vi "Nicolet 12 ICAI_gatefix2.vi"(3 "?":u16(ring)=9 items=["16", "32", "64", "128", "256", "512", "1024", "2048", "4096", "8192", "16384", "32768", "65536", "131072", "262144", "524288 (one channel)", ""], 5 "Sample Duration (sec)":u32(knob)=24 scale=1.0..33.0) -> (0 "Waveform Graph":waveform(dbl)[](graph)=[{"t0"=timestamp(0 s since 1904-01-01), "dt"=0.0001220703125, "Y"=array[40960 elements]}, {"t0"=timestamp(0 s since 1904-01-01), "dt"=0.0001220703125, "Y"=array[40960 elements]}], 2 "data":dbl[][](array[numeric]) format="%0.2f", 8 "points":i32=40960)   [LabVIEW 2010]
doc: "I. Description:\nThis example demonstrates how to acquire a finite amount of data (Waveform) using the DAQ device's internal clock, started by an analog edge condition.\n\nII. Instructions for Running:\n1. Select the physical channel to correspond to where your signal is input on the DAQ device.\n2. Enter the minimum and maximum voltage range.\nNote: For better accuracy try to match the input range to the expected voltage level of the measured signal.\n3. Set the number of samples to acquire per channel.\n4. Set the rate of the acquisition\nNote: The rate should be AT LEAST twice as fast as the maximum frequency component of the signal being acquired.\n5. Set the source of the start trigger. By default this is PFI0\n6. Set the slope and level of desired analog edge condition.\n\nIII. Block Diagram Steps:\n1. Create an empty task.\n2. Create an analog input voltage channel.\n3. Set the rate for the sample clock. Additionally, define the sample mode to be finite.\n4. Define the parameters for an Analog Slope Start Trigger.\n5. Call the Start VI to start the acquisition.\n6. Read all of the data.\n7. Stop the Analog Input Task.\n8. Call the Clear Task VI to clear the Task.\n9. Use the popup dialog box to display an error if any\nIV. I/O Connections Overview:\nMake sure your signal input terminal matches the Physical Channel I/O Control. In this case wire your signal to the ai0 pin on your DAQ Device."
uses:
  programs/Detection/200262.llb/Trigger Select.ctl
  <vilib>/Utility/error.llb/DialogType.ctl
  <vilib>/DAQmx/write.llb/DAQmx Write (Analog DBL 1Chan 1Samp).vi
  <vilib>/DAQmx/read.llb/DAQmx Read (Analog 2D DBL NChan NSamp).vi
  <vilib>/DAQmx/create/channels.llb/DAQmx Create Channel (AO-Voltage-Basic).vi
  <vilib>/daqmx/miscellaneous.llb/DAQmx Fill In Error Info.vi
  <vilib>/DAQmx/create/channels.llb/DAQmx Create Channel (AI-Voltage-Basic).vi
  <vilib>/DAQmx/configure/timing.llb/DAQmx Timing (Sample Clock).vi
  <vilib>/DAQmx/configure/trigger.llb/DAQmx Start Trigger (Analog Edge).vi
  <vilib>/DAQmx/configure/trigger.llb/DAQmx Reference Trigger (Digital Edge).vi
  <vilib>/measure/maspectr.llb/FFT Power Spectral Density for 1 Chan.vi
  <vilib>/measure/NI_MAPro.lvlib
  Program Files/National Instruments/LabVIEW 2010/resource/objmgr/daqmx.rc
panel:
  out "size(s)":i32[](array[numeric])
  in  "CAI/ICAI":bool=TRUE
  in  "?":path=path "C:/Users/Cardenas/Desktop/7_01/7_01_380fringe371mvmid_lockedat330.txt"
  in  "Path":path=path "C:/Users/Cardenas/Desktop/7_03/a6_200ms_span.txt"
  out "Time":dbl=5.5
  out "points pretriger":dbl=4096.0
  in  "Iterations to Average":i32=30
  in  "Sample Rate Hz":bool
  out "Cursor Time Selected":dbl=0.22413589186805782
  out "Cursor Peak to Peak Voltage":dbl=0.01024955436720143
  in  "Save Average To File":bool
  out "Pretrigger Samples":dbl=4096.0
  out "Seconds Per Division":dbl=0.1
  out "Posttrigger Samples Captured":dbl=40960.0
  in  "Voltage Offset":dbl(knob) scale=-2.0..2.0
  in  "Average / Live Display":bool
  in  "Seconds  Per Division":u32(knob) min=1 max=1 step=1 scale=0.0..15.0
  out "Samples Averaged":i32=3
  in  "?":bool=TRUE
  in  "Volts Per Division":dbl(knob)=0.5 scale=0.005..5.0
  in  "Pretrigger Duration (%)":dbl(knob)=0.1 min=0.0 max=2.0 step=1.0 scale=0.05..0.95
  in  "Analog Source":string="APFI0"
  in  "Digital External TTL Source":tag="/Dev1/PFI0"
  in  "Trigger Type":T1=enum."Analog Edge"
  in  "Analog Edge Level":dbl=-0.1 format="%0.2f"
  in  "Edge":i32(ring)=10280 items=["Rising"=10280, "Falling"=10171]
  in  "Physical Channel":tag="Dev1/ai22, Dev1/ai23" caption="Physical Channels"
  out "Sampling Iterations":i32=2
  in  "Maximum  Voltage":dbl=10.0
  in  "Minimum Voltage":dbl=-10.0
  out "Sampling Rate":i32=8192 caption="Sample Rate (Hz)"
  in  "stop":bool
  # "Channel\nConfiguration"
  # "Triggering Parameters"
  # "Voltage Parameters"
  # "TTL Trigger Options"
  # "Timing Parameters"
  # "External  Trigger Options"
  # "Storage Options"
  # "Nicolet 8.vi*If X scale markers are not drawn:\nRight click the waveform diagram -> select X axis -> marker spacing -> set to arbitrary AFTER\nsetting the correct seconds per division"
  # "CAI / ICAI"
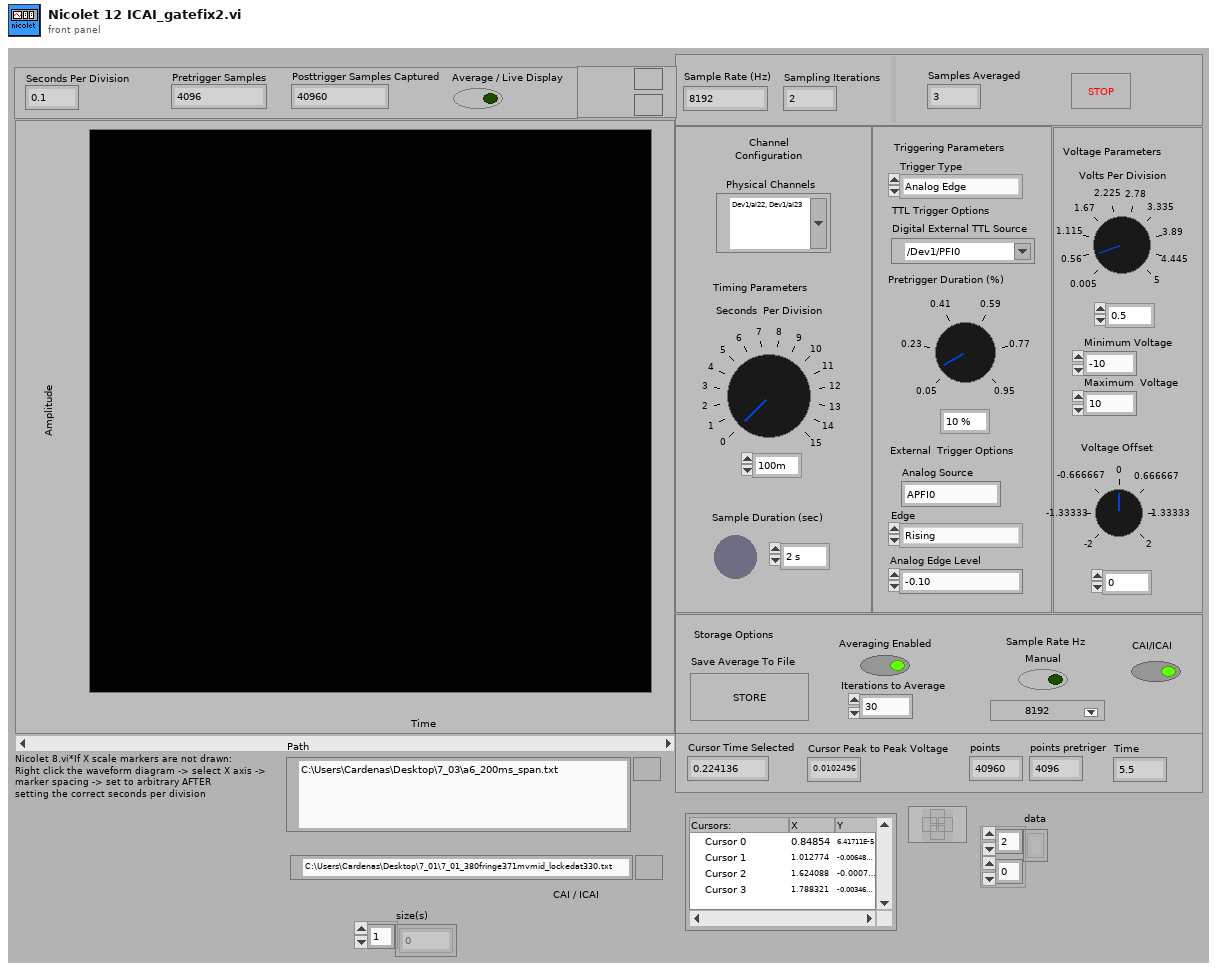
[diagram p1: front panel]
types:
  T1 = typedef "Trigger Select.ctl" = enum16{"None", "Analog Edge", "Digital Edge"}
  T2 = typedef "DialogType.ctl" = u16
  T3 = typedef "LVCursorListTypeDef.ctl" = cluster{"Name":string, "Color":u32, "Style":u8, "Point Style":u8, "Name Visible":bool, "Allow Drag":bool, "Cursor Mode":u32, "Plot":i32, "Index":i32, "Position":cluster{"X":dbl, "Y":dbl}, "X Scale":u32, "Y Scale":u32, "Watch Plots":i32[], "Watch All Plots":bool, "Plot Area":i32, "Label Offset":cluster{"X":dbl, "Y":dbl}}[]
  T4 = cluster{"Name":string, "Color":u32, "Style":u8, "Point Style":u8, "Name Visible":bool, "Allow Drag":bool, "Cursor Mode":u32, "Plot":i32, "Index":i32, "Position":cluster{"X":dbl, "Y":dbl}, "X Scale":u32, "Y Scale":u32, "Watch Plots":i32[], "Watch All Plots":bool, "Plot Area":i32, "Label Offset":cluster{"X":dbl, "Y":dbl}}
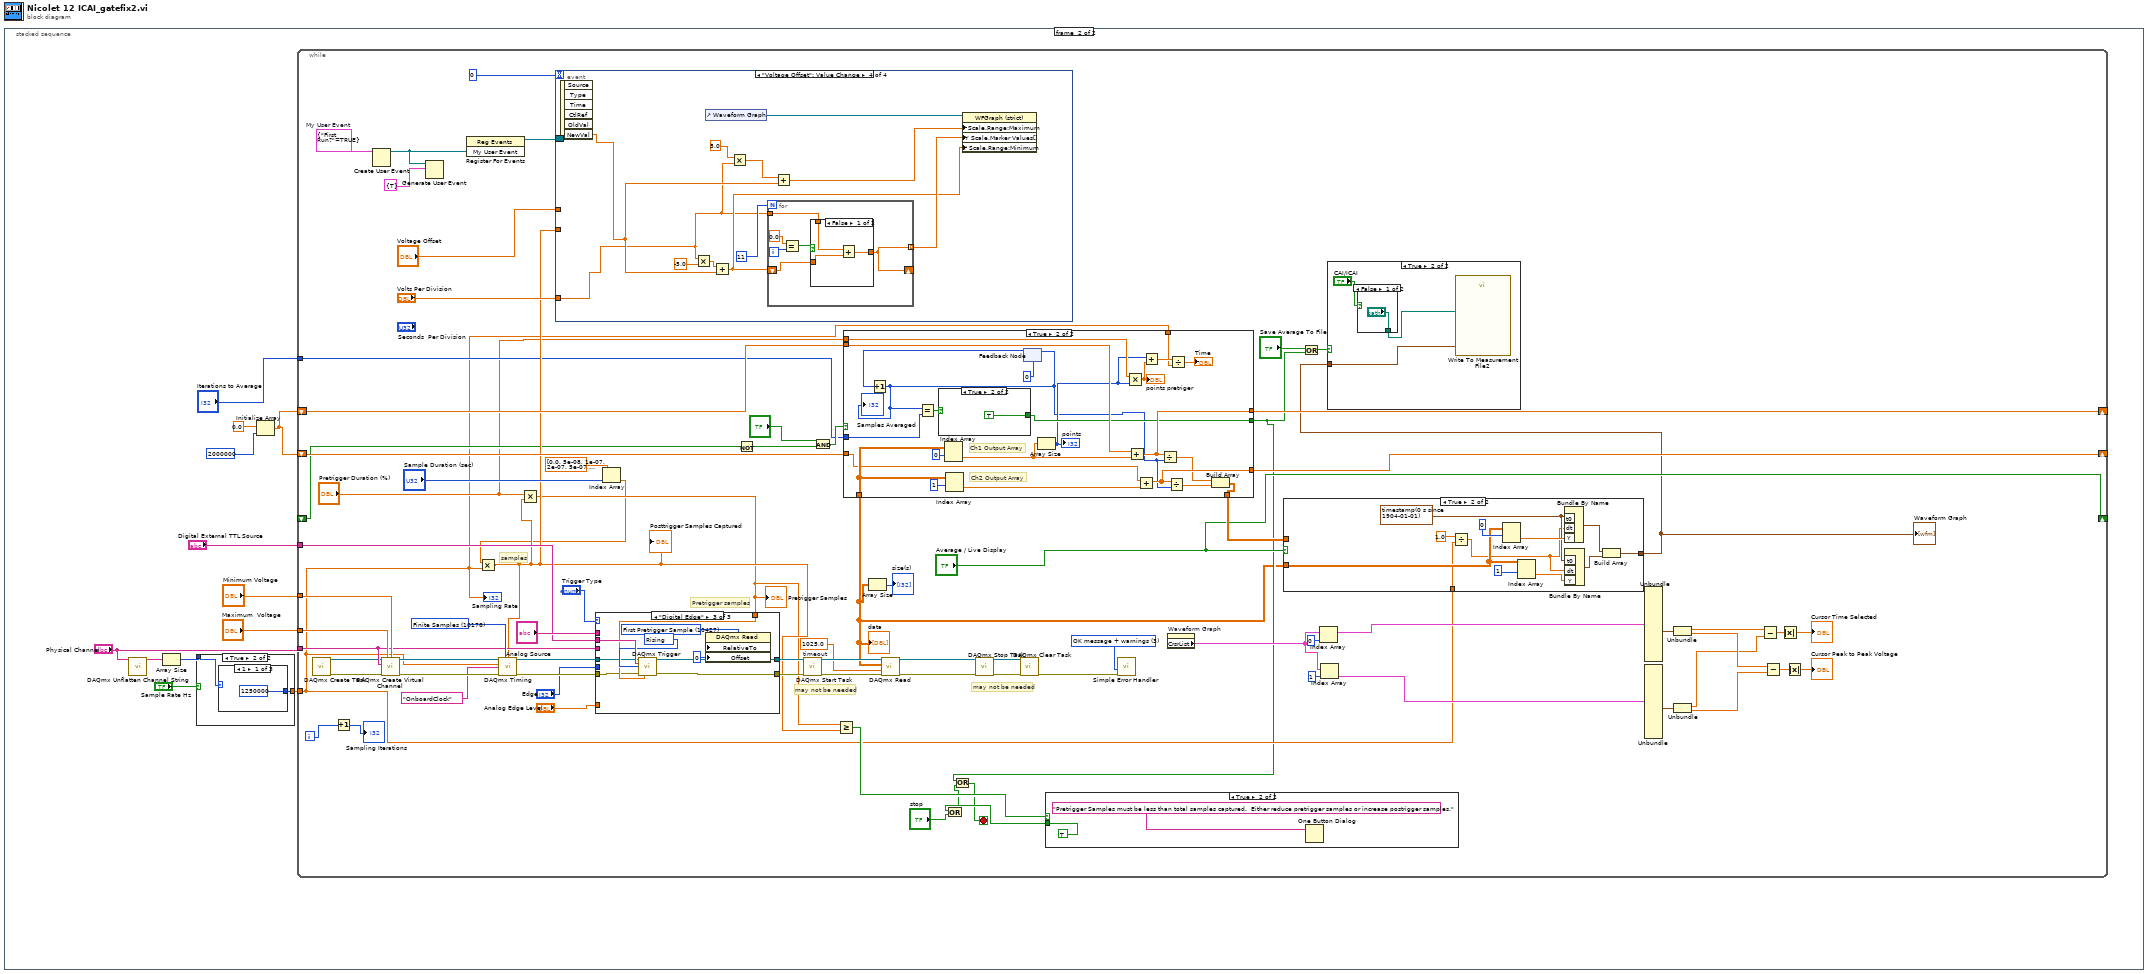
[diagram p0: block diagram]
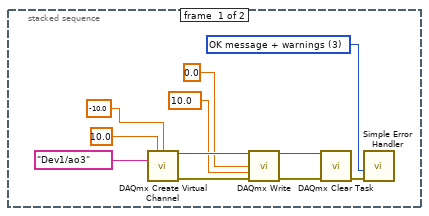
[diagram p2: hidden frame]
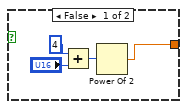
[diagram p3: hidden frame]
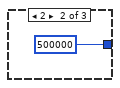
[diagram p4: hidden frame]
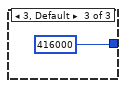
[diagram p5: hidden frame]
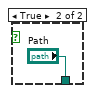
[diagram p7: hidden frame]
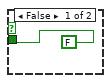
[diagram p8: hidden frame]
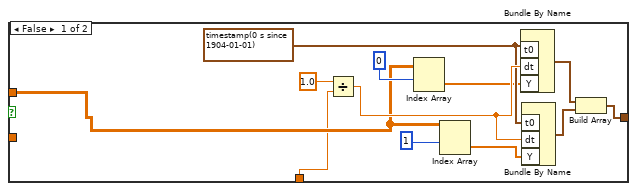
[diagram p9: hidden frame]
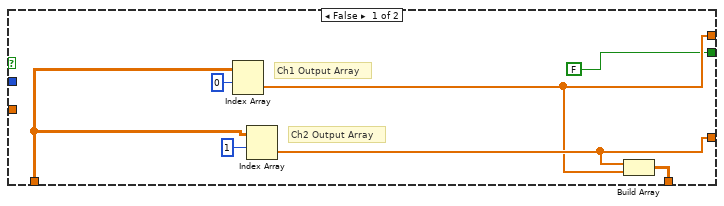
[diagram p10: hidden frame]
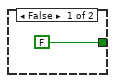
[diagram p11: hidden frame]
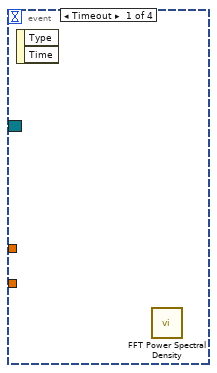
[diagram p12: hidden frame]
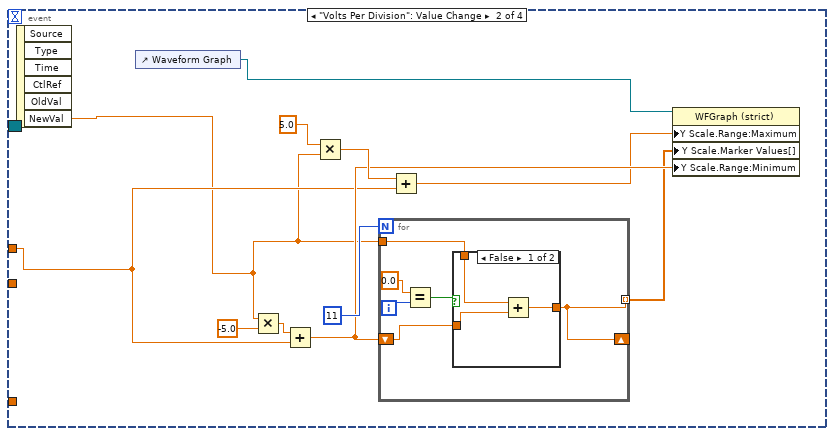
[diagram p13: hidden frame]
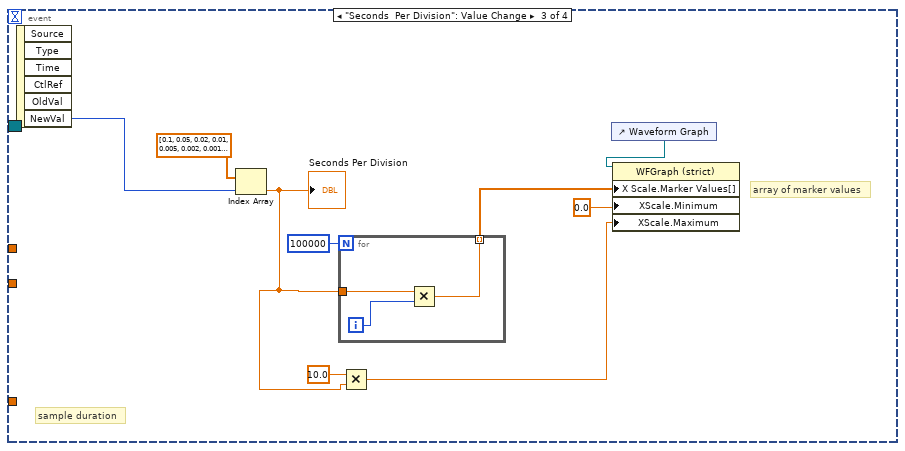
[diagram p15: hidden frame]
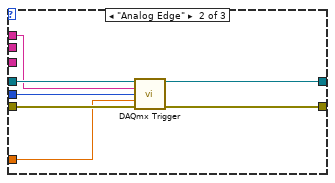
[diagram p18: hidden frame]
diagram:
  n1 = stacked-sequence {
    frame #0 {
      w4 = T2 3 items=["no dialog", "OK message", "continue or stop message", "OK message + warnings", "continue/stop + warnings"] ("type of dialog (OK msg:1)")
      n2 = call-poly <vilib>:"DAQmx Create Virtual Channel.vi"("maximum value"=10.0 ("Maximum Value"), "minimum value"=-10.0 ("Minimum Value"), "physical channels"=tag "Dev1/ao3" ("Physical Channel")) -> ("task out"=w7:refnum<k21>, "error out"=w8:errorcluster)  [unwired: 6 in, 5 out]
      n3 = call-poly <vilib>:"DAQmx Write.vi"("task/channels in"=w7, "data"=0.0 ("Voltage Output"), "timeout"=10.0, "error in"=w8) -> ("task out"=w2:refnum<k21>, "error out"=w3:errorcluster)  [unwired: 1 in, 9 out]
      n4 = call <vilib>:"DAQmx Clear Task.vi"("task in"=w2, "error in"=w3) -> ("error out"=w1:errorcluster)  [unwired: 13 out]
      n5 = call <vilib>:"Simple Error Handler.vi"("type of dialog (OK msg:1)"=w4, "error in (no error)"=w1) -> ()  [unwired: 8 out]
    }
    frame #1 {
      n6 = call <vilib>:"DAQmx Unflatten Channel String.vi"("names in"="Physical Channel") -> ("names out"=w19:string[])  [unwired: 1 in, 13 out]
      n7 = Array Size(array=w19) -> (size(s)=w17:i32)
      n8 = case shown="True" "Sample Rate Hz" {
        tunnel: [w25 w29] -> w18
        tunnel: w17 -> [_ w28]
        frame False {
          n9 = Add(x=4, y="?") -> (x+y=w26:i32)
          n10 = Power Of 2(x=w26) -> (2^x=w25:dbl)
        }
        frame True {
          n11 = case shown="1" w28 {
            tunnel: [1250000 500000 416000] -> w29
            frame 1 {
            }
            frame 2 {
            }
            frame 3, Default {
            }
          }
        }
      }
      n12 = Initialize Array(0.0, 2000000) -> (w12:dbl[])
      n13 = while {
        tunnel: "Minimum Voltage" -> [w93]
        tunnel: "Maximum  Voltage" -> [w92]
        tunnel: "Physical Channel" -> [w91]
        tunnel: "Digital External TTL Source" -> [w89]
        shift-right: [w83] -> _
        shift-left: w12 -> [w82]
        shift-right: [w78] -> _
        shift-left: w12 -> [w77]
        tunnel: w18 -> [w40]
        shift-right: ["Average / Live Display"] -> _
        shift-left: _ -> [w50]
        tunnel: "Iterations to Average" -> [w42]
        i -> [w36]
        stop <- w39 stop-if-true
        w88 = cluster{"First Run?":bool} {"First Run?"=TRUE}  # My User Event
        w108 = T2 3 items=["no dialog", "OK message", "continue or stop message", "OK message + warnings", "continue/stop + warnings"] ("type of dialog (OK msg:1)")
        w105 = 1025.0  # timeout
        w103 = 10178 items=["Finite Samples"=10178, "Continuous Samples"=10123] ("sample mode")
        # "samples"
        # "may not be needed"
        # "may not be needed"
        # "Pretrigger samples"
        n14 = call <vilib>:"DAQmx Create Task.vi"() -> ("task out"=w81:refnum<k21>, "error out"=w80:errorcluster)  [unwired: 5 in, 9 out]
        n15 = Increment(x=w36) -> (x+1=→"Sampling Iterations":i32)
        n16 = Create User Event(user event datatype=w88) -> (user event=w86:refnum<user-event>)  [unwired: 1 in, 1 out]
        n17 = call-poly <vilib>:"DAQmx Create Virtual Channel.vi"("task in"=w81, "maximum value"=w92, "minimum value"=w93, "physical channels"=w91, "error in"=w80) -> ("task out"=w104:refnum<k21>, "error out"=w112:errorcluster)  [unwired: 4 in, 5 out]
        n18 = Generate User Event(user event=w86, event data cluster=cluster{"First Run?":bool} {"First Run?"=TRUE} ("event data")) -> ()  [unwired: 1 in, 2 out]
        n19 = register-events(w86) -> (reference out=w84:refnum<event-registration>)  [unwired: 2 in, 1 out]
        n20 = Index Array(array=dbl[] [0.0, 5e-08, 1e-07, 2e-07, 5e-07, 1e-06, 2e-06, 5e-06, 1e-05, 2e-05, 5e-05, 0.0001, 0.0002, 0.0005, 0.001, 0.002, 0.005, 0.01, 0.02, 0.05, 0.1, 0.2, 0.5, 1.0, 2.0, 5.0, 10.0, 16.5, 32.5, 65.0, 129.0, 257.0, 513.0, 1025.0], index="Sample Duration (sec)") -> (element=w47:dbl)
        n21 = Multiply(x=w47, y=w40) -> (x*y=w69:dbl)
        "Posttrigger Samples Captured" <- w69
        n22 = call-poly <vilib>:"DAQmx Timing.vi"("task/channels in"=w104, "sample mode"=w103, "samples per channel"=w69, "rate"=w40, "source"=tag "OnboardClock", "error in"=w112) -> ("task out"=w98:refnum<k21>, "error out"=w96:errorcluster)  [unwired: 1 in, 7 out]
        n23 = Multiply(x="Pretrigger Duration (%)", y=w69) -> (x*y=w68:dbl)
        "Pretrigger Samples" <- w68
        n24 = event shown="[3] \"Voltage Offset\": Value Change" {
          selector: w84 -> [_ _ _ _]
          dyn-events: _ -> [_ _ _ _]
          timeout: 0 -> [_ _ _ _]
          tunnel: w69 -> [_ _ _ _]
          tunnel: "Voltage Offset" -> [_ w180 _ _]
          tunnel: "Volts Per Division" -> [_ _ _ w212]
          event Timeout {
            n25 = event-data() -> ()  [unwired: 3 out]
            n26 = call-poly <vilib>:"FFT Power Spectral Density.vi"() -> ()  [unwired: 6 in, 6 out]
          }
          event "Volts Per Division": Value Change {
            n27 = event-data() -> ("NewVal"=w179:dbl)  [unwired: 6 out]
            n28 = control-ref of="Waveform Graph"() -> (w178:refnum<vi>)
            n29 = Multiply(x=w179, y=-5.0) -> (x*y=w185:dbl)
            n30 = Add(x=w185, y=w180) -> (x+y=w183:dbl)
            n31 = Multiply(x=5.0, y=w179) -> (x*y=w184:dbl)
            n32 = for {
              N: 11 -> [_]
              tunnel: w179 -> [w194]
              tunnel: [w193] -> w181 mode=indexing
              shift-right: [w193] -> _
              shift-left: w183 -> [w191]
              i -> [w189]
              n33 = Equal?(x=0.0, y=w189) -> (x = y?=w192:bool)
              n34 = case shown="False" w192 {
                tunnel: w194 -> [w197 _]
                tunnel: w191 -> [w196 w198]
                tunnel: [w195 w198] -> w193
                frame False {
                  n35 = Add(x=w197, y=w196) -> (x+y=w195:dbl)
                }
                frame True {
                }
              }
            }
            n36 = Add(x=w184, y=w180) -> (x+y=w182:dbl)
            n37 = property on="Property Node" class="WFGraph (strict)"(reference=w178, "Y Scale.Range:Maximum"=w182, "Y Scale.Marker Values[]"=w181, "Y Scale.Range:Minimum"=w183) -> ()  [unwired: 1 in, 2 out]
          }
          event "Seconds  Per Division": Value Change {
            # "sample duration"
            # "array of marker values"
            n38 = event-data() -> ("NewVal"=w206:u32)  [unwired: 6 out]
            n39 = Index Array(array=dbl[] [0.1, 0.05, 0.02, 0.01, 0.005, 0.002, 0.001, 0.0005, 0.0002, 0.0001, 5e-05, 2e-05, 1e-05, 5e-06, 2e-06, 1e-06], index=w206) -> (element=w200:dbl)
            "Seconds Per Division" <- w200
            n40 = for {
              N: 100000 -> [_]
              tunnel: w200 -> [w209]
              tunnel: [w208] -> w202 mode=indexing
              i -> [w210]
              n41 = Multiply(x=w209, y=w210) -> (x*y=w208:dbl)
            }
            n42 = Multiply(x=10.0, y=w200) -> (x*y=w199:dbl)
            n43 = control-ref of="Waveform Graph"() -> (w204:refnum<vi>)
            n44 = property on="Property Node" class="WFGraph (strict)"(reference=w204, "X Scale.Marker Values[]"=w202, "XScale.Minimum"=0.0 ("x"), "XScale.Maximum"=w199) -> ()  [unwired: 1 in, 2 out]
          }
          event "Voltage Offset": Value Change {
            n45 = event-data() -> ("NewVal"=w213:dbl)  [unwired: 6 out]
            n46 = Multiply(x=w212, y=-5.0) -> (x*y=w220:dbl)
            n47 = control-ref of="Waveform Graph"() -> (w211:refnum<vi>)
            n48 = Add(x=w220, y=w213) -> (x+y=w214:dbl)
            n49 = Multiply(x=5.0, y=w212) -> (x*y=w221:dbl)
            n50 = for {
              N: 11 -> [_]
              tunnel: w212 -> [w227]
              tunnel: [w226] -> w215 mode=indexing
              shift-right: [w226] -> _
              shift-left: w214 -> [w224]
              i -> [w222]
              n51 = Equal?(x=0.0, y=w222) -> (x = y?=w225:bool)
              n52 = case shown="False" w225 {
                tunnel: w227 -> [w230 _]
                tunnel: w224 -> [w229 w231]
                tunnel: [w228 w231] -> w226
                frame False {
                  n53 = Add(x=w230, y=w229) -> (x+y=w228:dbl)
                }
                frame True {
                }
              }
            }
            n54 = Add(x=w221, y=w213) -> (x+y=w216:dbl)
            n55 = property on="Property Node" class="WFGraph (strict)"(reference=w211, "Y Scale.Range:Maximum"=w216, "Y Scale.Marker Values[]"=w215, "Y Scale.Range:Minimum"=w214) -> ()  [unwired: 1 in, 2 out]
          }
        }
        n56 = case shown="\"Digital Edge\"" "Trigger Type" {
          tunnel: w98 -> [w233 w236 w247]
          tunnel: [w233 w238 w243] -> w97
          tunnel: w96 -> [w232 w240 w245]
          tunnel: [w232 w237 w250] -> w95
          tunnel: w91 -> [_ _ _]
          tunnel: "Analog Edge Level" -> [_ w239 _]
          tunnel: "Analog Source" -> [_ w235 _]
          tunnel: w89 -> [_ _ w249]
          tunnel: w68 -> [_ _ w246]
          tunnel: "Edge" -> [_ w234 _]
          frame "None", Default {
          }
          frame "Analog Edge" {
            n57 = call-poly <vilib>:"DAQmx Trigger.vi"("task/channels in"=w236, "source"=w235, "slope"=w234, "level"=w239, "error in"=w240) -> ("task out"=w238:refnum<k21>, "error out"=w237:errorcluster)  [unwired: 9 out]
          }
          frame "Digital Edge" {
            w241 = 10427 items=["First Sample"=10424, "Current Read Position"=10425, "Reference Trigger"=10426, "First Pretrigger Sample"=10427, "Most Recent Sample"=10428] ("RelativeTo")
            w248 = 10280 items=["Rising"=10280, "Falling"=10171] ("edge")
            n58 = call-poly <vilib>:"DAQmx Trigger.vi"("task/channels in"=w247, "source"=w249, "edge"=w248, "error in"=w245, "pretrigger samples per channel"=w246) -> ("task out"=w244:refnum<k21>, "error out"=w250:errorcluster)  [unwired: 9 out]
            n59 = property class="DAQmx Read"(reference=w244, "RelativeTo"=w241, "Offset"=0) -> (reference out=w243:refnum<k21>)  [unwired: 1 in, 1 out]
          }
        }
        n60 = Not(x=w50) -> (.not. x?=w49:bool)
        n61 = call <vilib>:"DAQmx Start Task.vi"("task/channels in"=w97, "error in"=w95) -> ("task out"=w106:refnum<k21>, "error out"=w111:errorcluster)  [unwired: 12 out]
        n62 = And(x="?", y=w49) -> (x .and. y?=w48:bool)
        n63 = Greater Or Equal?(x=w68, y=w69) -> (x >= y?=w72:bool)
        n64 = call-poly <vilib>:"DAQmx Read.vi"("task/channels in"=w106, "timeout"=w105, "error in"=w111) -> ("task out"=w102:refnum<k21>, "data"=w34:dbl[][], "error out"=w101:errorcluster)  [unwired: 1 in, 9 out]
        "data" <- w34
        n65 = case shown="True" w48 {
          tunnel: w34 -> [w149 w175]
          tunnel: [w147 w170] -> w83
          tunnel: w82 -> [_ w168]
          tunnel: [w148 w167] -> w78
          tunnel: w77 -> [_ w166]
          tunnel: [w146 w163] -> w67
          tunnel: [FALSE w161] -> w37
          tunnel: w42 -> [_ w159]
          tunnel: "Pretrigger Duration (%)" -> [_ w158]
          tunnel: w40 -> [_ w154]
          frame False {
            # "Ch2 Output Array"
            # "Ch1 Output Array"
            n66 = Index Array(array=w149, index (row)=0 ("disabled index (col)")) -> (element=w147:dbl[])  [unwired: 1 in]
            n67 = Index Array(array=w149, index (row)=1 ("disabled index (col)")) -> (element=w148:dbl[])  [unwired: 1 in]
            n68 = Build Array(w148, w147) -> (w146:dbl[][])
          }
          frame True {
            # "Ch2 Output Array"
            # "Ch1 Output Array"
            n69 = Index Array(array=w175, index (row)=0 ("disabled index (col)")) -> (element=w162:dbl[])  [unwired: 1 in]
            n70 = Index Array(array=w175, index (row)=1 ("disabled index (col)")) -> (element=w169:dbl[])  [unwired: 1 in]
            n71 = feedback #1(0) -> (w171:i32)
            n72 = Increment(x=w171) -> (x+1=w152:i32)
            "Samples Averaged" <- w152
            n73 = Equal?(x=w152, y=w159) -> (x = y?=w160:bool)
            n74 = case shown="True" w160 {
              tunnel: [FALSE TRUE] -> w161
              frame False {
              }
              frame True {
              }
            }
            n75 = feedback-in #1(w152) -> ()
            n76 = Array Size(array=w162) -> (size(s)=w157:i32)
            "points" <- w157
            n77 = Multiply(x=w158, y=w157) -> (x*y=w156:dbl)
            "points pretriger" <- w156
            n78 = Add(x=w168, y=w162) -> (x+y=w170:dbl[])
            n79 = Add(x=w166, y=w169) -> (x+y=w167:dbl[])
            n80 = Add(x=w157, y=w156) -> (x+y=w155:dbl)
            n81 = Divide(x=w170, y=w152) -> (x/y=w165:dbl[])
            n82 = Divide(x=w167, y=w152) -> (x/y=w164:dbl[])
            n83 = Divide(x=w155, y=w154) -> (x/y=→"Time":dbl)
            n84 = Build Array(w165, w164) -> (w163:dbl[][])
          }
        }
        n85 = Array Size(array=w34) -> (size(s)=→"size(s)":i32[])
        n86 = call <vilib>:"DAQmx Stop Task.vi"("task/channels in"=w102, "error in"=w101) -> ("task out"=w107:refnum<k21>, "error out"=w110:errorcluster)  [unwired: 12 out]
        n87 = call <vilib>:"DAQmx Clear Task.vi"("task in"=w107, "error in"=w110) -> ("error out"=w109:errorcluster)  [unwired: 13 out]
        n88 = case shown="True" w72 {
          tunnel: [FALSE TRUE] -> w70
          frame False {
          }
          frame True {
            n89 = One Button Dialog(message="Pretrigger Samples must be less than total samples captured.  Either reduce pretrigger samples or increase postrigger samples.") -> ()  [unwired: 2 out]
          }
        }
        n90 = Or(x=w70, y="stop") -> (x .or. y?=w38:bool)
        n91 = Or(x=w37, y=w38) -> (x .or. y?=w39:bool)
        n92 = call <vilib>:"Simple Error Handler.vi"("type of dialog (OK msg:1)"=w108, "error in (no error)"=w109) -> ()  [unwired: 8 out]
        n93 = property on="Waveform Graph" class="WFGraph (strict)"() -> ("CrsrList"=w46:T3)  [unwired: 2 in, 2 out]
        n94 = case shown="True" "Average / Live Display" {
          tunnel: w34 -> [_ w141]
          tunnel: [w123 w133] -> w45
          tunnel: w67 -> [w125 _]
          tunnel: w40 -> [w124 w137]
          frame False {
            w130 = timestamp(0 s since 1904-01-01) ("t0")
            n95 = Divide(x=1.0, y=w124) -> (x/y=w132:dbl)
            n96 = Index Array(array=w125, index (row)=0 ("disabled index (col)")) -> (element=w126:dbl[])  [unwired: 1 in]
            n97 = Index Array(array=w125, index (row)=1 ("disabled index (col)")) -> (element=w129:dbl[])  [unwired: 1 in]
            n98 = Bundle By Name("t0"=w130, "dt"=w132, "Y"=w126) -> (w121:waveform(dbl))  [unwired: 1 out]
            n99 = Bundle By Name("t0"=w130, "dt"=w132, "Y"=w129) -> (w122:waveform(dbl))  [unwired: 1 out]
            n100 = Build Array(w121, w122) -> (w123:waveform(dbl)[])
          }
          frame True {
            w139 = timestamp(0 s since 1904-01-01) ("t0")
            n101 = Divide(x=1.0, y=w137) -> (x/y=w136:dbl)
            n102 = Index Array(array=w141, index (row)=0 ("disabled index (col)")) -> (element=w144:dbl[])  [unwired: 1 in]
            n103 = Index Array(array=w141, index (row)=1 ("disabled index (col)")) -> (element=w140:dbl[])  [unwired: 1 in]
            n104 = Bundle By Name("t0"=w139, "dt"=w136, "Y"=w144) -> (w134:waveform(dbl))  [unwired: 1 out]
            n105 = Bundle By Name("t0"=w139, "dt"=w136, "Y"=w140) -> (w135:waveform(dbl))  [unwired: 1 out]
            n106 = Build Array(w134, w135) -> (w133:waveform(dbl)[])
          }
        }
        "Waveform Graph" <- w45
        n107 = Or(x="Save Average To File", y=w37) -> (x .or. y?=w44:bool)
        n108 = Index Array(array=w46, index=0) -> (element=w64:T4)
        n109 = Index Array(array=w46, index=1) -> (element=w63:T4)
        n110 = case shown="True" w44 {
          tunnel: w45 -> [_ w115]
          frame False {
          }
          frame True {
            n111 = case shown="False" "CAI/ICAI" {
              tunnel: ["?" "Path"] -> w114
              frame False {
              }
              frame True {
              }
            }
            n112 = call "Write To Measurement File2"("Signals"=w115, "Filename"=w114) -> ()  [unwired: 15 in, 3 out]
          }
        }
        n113 = Unbundle(w64) -> ("Position"=w62:cluster{"X":dbl, "Y":dbl})  [unwired: 15 out]
        n114 = Unbundle(w63) -> ("Position"=w61:cluster{"X":dbl, "Y":dbl})  [unwired: 15 out]
        n115 = Unbundle(w62) -> ("X"=w56:dbl, "Y"=w60:dbl)
        n116 = Unbundle(w61) -> ("X"=w54:dbl, "Y"=w59:dbl)
        n117 = Subtract(x=w56, y=w54) -> (x-y=w55:dbl)
        n118 = Subtract(x=w60, y=w59) -> (x-y=w58:dbl)
        n119 = Absolute Value(x=w55) -> (abs(x)=→"Cursor Time Selected":dbl)
        n120 = Absolute Value(x=w58) -> (abs(x)=→"Cursor Peak to Peak Voltage":dbl)
        "Sampling Rate" <- w40
      }
    }
  }
